vi "testMapSensorIdToName.vi"(8 "error in (no error)":errorcluster) -> (0 "error out":errorcluster)   [LabVIEW 2016]
doc: "Test to map the sensor Id to sensor name."
uses:
  ZTAAC/ZTAAC.lvclass
  StrictDef/InstName.ctl
  <vilib>/addons/_JKI Toolkits/Caraya/classes/Test/Test.lvclass
  <vilib>/addons/_JKI Toolkits/Caraya/classes/Assert/Assert.lvclass
  OfcFunc.lvlib
panel:
  in  "ZTAAC.lvclass":refnum<class "ZTAAC.lvclass">
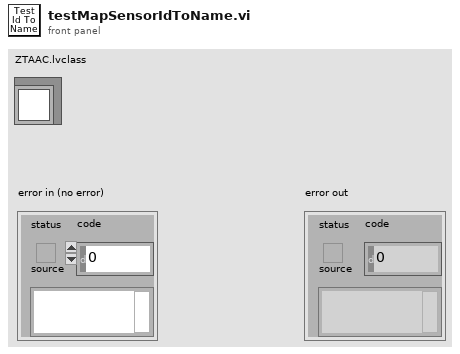
[diagram p1: front panel]
types:
  T1 = typedef "OfcFunc.lvlib/InstName.ctl" = enum16{"lsst", "comcam"}
  T2 = cluster{"Config Dir":path, "Inst Name":T1, "OptStateEsti Config File Name":string, "Mapping File Name":string, "Wavelength Table":string, "Intrinc Zk File Name":string, "y2 Corection File Name":string, "Index DOF File Name":string, "OptCtrl Config File Name":string, "State 0 File Name":string, "Weighting File Name":string, "PSSN Alpha File Name":string, "Authority Files":cluster{"Rigid Body Stroke File":string, "M1M3 Subsystem":cluster{"Mirror":string, "Actuatro Force File":string}, "M2 Subsystem":cluster{"Mirror":string, "Actuatro Force File":string}, "Num of Bending Mode":i32}, "Sensor Id to Name File Name":string, "Truncation Threshold":dbl, "Default Gain":dbl, "FWHM Threshold (arcsec)":dbl}
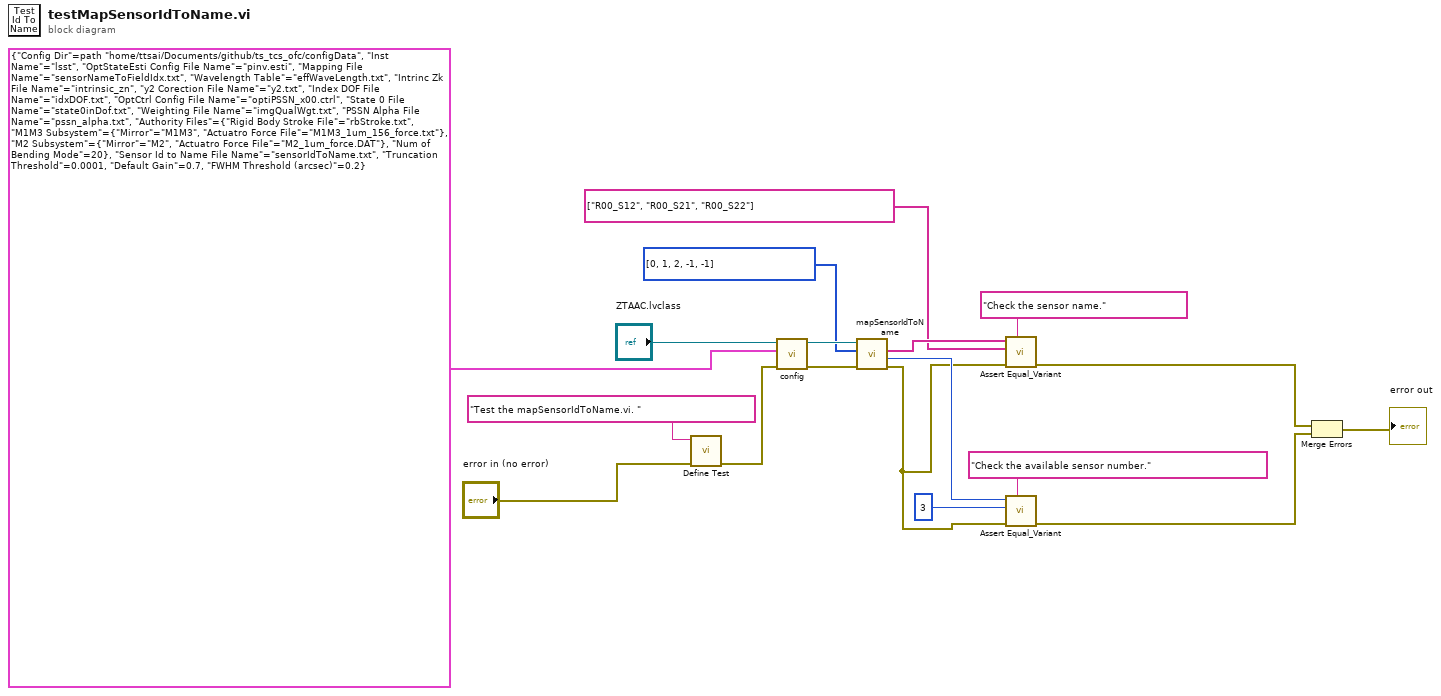
[diagram p0: block diagram]
diagram:
  n1 = call <vilib>:"Define Test.vi"("error in (no error)"="error in (no error)", "Label (VI Title)"="Test the mapSensorIdToName.vi. ") -> ("error out"=w15:errorcluster)  [unwired: 9 in]
  n2 = call "config.vi"("error in (no error)"=w15, "ZTAAC Configuration"=T2 {"Config Dir"=path "/home/ttsai/Documents/github/ts_tcs_ofc/configData", "Inst Name"=enum."lsst", "OptStateEsti Config File Name"="pinv.esti", "Mapping File Name"="sensorNameToFieldIdx.txt", "Wavelength Table"="effWaveLength.txt", "Intrinc Zk File Name"="intrinsic_zn", "y2 Corection File Name"="y2.txt", "Index DOF File Name"="idxDOF.txt", "OptCtrl Config File Name"="optiPSSN_x00.ctrl", "State 0 File Name"="state0inDof.txt", "Weighting File Name"="imgQualWgt.txt", "PSSN Alpha File Name"="pssn_alpha.txt", "Authority Files"={"Rigid Body Stroke File"="rbStroke.txt", "M1M3 Subsystem"={"Mirror"="M1M3", "Actuatro Force File"="M1M3_1um_156_force.txt"}, "M2 Subsystem"={"Mirror"="M2", "Actuatro Force File"="M2_1um_force.DAT"}, "Num of Bending Mode"=20}, "Sensor Id to Name File Name"="sensorIdToName.txt", "Truncation Threshold"=0.0001, "Default Gain"=0.7, "FWHM Threshold (arcsec)"=0.2}, "ZTAAC in"="ZTAAC.lvclass") -> ("error out"=w13:errorcluster, "ZTAAC out"=w14:refnum<class "ZTAAC.lvclass">)  [unwired: 7 in]
  n3 = call "mapSensorIdToName.vi"("error in (no error)"=w13, "Sensor Id"=i32[] [0, 1, 2, -1, -1], "ZTAAC in"=w14) -> ("error out"=w9:errorcluster, "Sensor Num"=w10:i32, "Sensor Name"=w8:string[])  [unwired: 5 in, 1 out]
  n4 = call <vilib>:"Assert Equal_Variant.vi"("Label"="Check the sensor name.", "error in (no error)"=w9, "Y"=string[] ["R00_S12", "R00_S21", "R00_S22"], "X"=w8) -> ("error out"=w6:errorcluster)  [unwired: 7 in]
  n5 = call <vilib>:"Assert Equal_Variant.vi"("Label"="Check the available sensor number.", "error in (no error)"=w9, "Y"=3, "X"=w10) -> ("error out"=w5:errorcluster)  [unwired: 7 in]
  n6 = Merge Errors(w6, w5) -> (→"error out":errorcluster)
